vi "TCP IP.vi"(1 "String 4":string, 2 "String 3":string, 3 "String 2":string, 4 "String 1":string) -> (0 "true":bool)   [LabVIEW 2022 SP3]
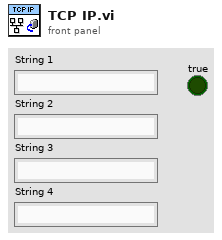
[diagram p1: front panel]
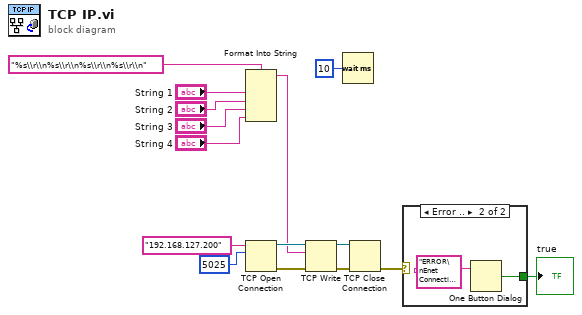
[diagram p0: block diagram]
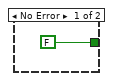
[diagram p2: hidden frame]
diagram:
  n1 = Format Into String(format string="%s\\r\\n%s\\r\\n%s\\r\\n%s\\r\\n", "String 1", "String 2", "String 3", "String 4") -> (resulting string=w8:string)  [unwired: 2 in, 1 out]
  n2 = TCP Open Connection(address="192.168.127.200", remote port or service name=u16 5025) -> (connection ID=w13:refnum<k5>, error out=w12:errorcluster)  [unwired: 3 in]
  n3 = TCP Write(connection ID=w13, data in=w8, error in (no error)=w12) -> (connection ID out=w15:refnum<k5>, error out=w14:errorcluster)  [unwired: 1 in, 1 out]
  n4 = Wait (ms)(milliseconds to wait=u32 10) -> ()  [unwired: 1 out]
  n5 = TCP Close Connection(connection ID=w15, error in (no error)=w14) -> (error out=w2:errorcluster)  [unwired: 1 in, 1 out]
  n6 = case shown="Error .." w2 {
    tunnel: [FALSE ("true") w17] -> w1
    frame No Error {
    }
    frame Error {
      n7 = One Button Dialog(message="ERROR\nEnet Connection ") -> (true=w17:bool)  [unwired: 1 in]
    }
  }
  "true" <- w1
